vi "Get Event Reg.vi"(8 "error in (no error)":errorcluster, 11 "2DArrayManager in":refnum<class "2DArrayManager.lvclass">) -> (0 "error out":errorcluster, 2 "Event Reg":refnum<event-registration>, 3 "2DArrayManager out":refnum<class "2DArrayManager.lvclass">)   [LabVIEW 2020, in "OOPanel.lvlib" / "2DArrayManager.lvclass"]
uses:
  2DArrayManager.lvclass
  2DArrayManager.lvclass/2DArrayManager.ctl
  2D Position.ctl
  2D Index.ctl
  Events.ctl
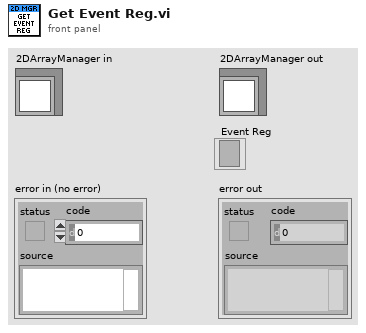
[diagram p1: front panel]
types:
  T1 = typedef "OOPanel.lvlib/2DArrayManager.lvclass/Event Reg Ref.ctl" = cluster{"Last Update Ticks ms":u32, "Event Reg":refnum<event-registration>}
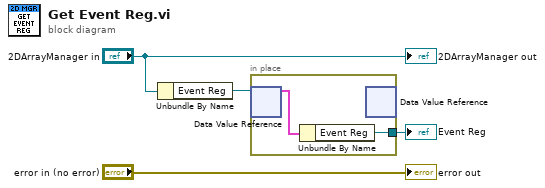
[diagram p0: block diagram]
diagram:
  n1 = Unbundle By Name("2DArrayManager in") -> ("Event Reg"=w3:refnum<data-value>)
  n2 = in-place {
    in-place-border: [w5] -> w1
    n3 = in-place-dvr #1(w3) -> (w6:T1)  [unwired: 1 out]
    n4 = Unbundle By Name(w6) -> ("Event Reg"=w5:refnum<event-registration>)
    n5 = in-place-dvr #1() -> ()  [unwired: 1 in, 2 out]
  }
  "Event Reg" <- w1
  "error out" <- "error in (no error)"
  "2DArrayManager out" <- "2DArrayManager in"
